vi "Open VIRef in Library App Context.vi"(8 "error in (no error)":errorcluster, 10 "vi path":path, 11 "library in":refnum<vi>) -> (0 "error out":errorcluster, 2 "vi":refnum<vi>, 3 "library out":refnum<vi>)   [LabVIEW 2019, in "gRPC Template Creation Utility.lvlib"]
uses:
  gRPC Template Creation Utility.lvlib
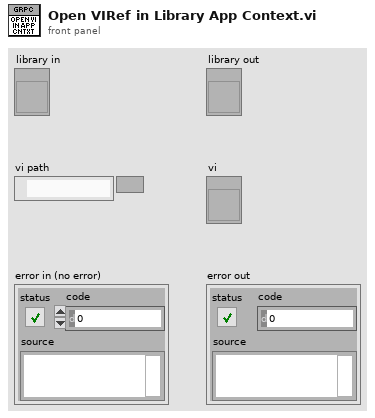
[diagram p1: front panel]
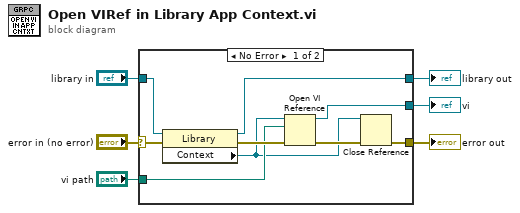
[diagram p0: block diagram]
diagram:
  n1 = case shown="No Error" "error in (no error)" {
    selector: "error in (no error)" -> [w11 w16]
    tunnel: "library in" -> [w12 w17]
    tunnel: [w14 w17] -> w5
    tunnel: [w8 w16] -> w4
    tunnel: [w15 _] -> w2
    tunnel: "vi path" -> [w10 _]
    frame No Error {
      n2 = property class="Library"(reference=w12, error in=w11) -> (reference out=w14:refnum<vi>, error out=w13:errorcluster, "Context"=w7:refnum<vi>)
      n3 = Open VI Reference(application reference (local)=w7, vi path=w10, error in (no error)=w13) -> (vi reference=w15:refnum<vi>, error out=w9:errorcluster)  [unwired: 3 in]
      n4 = Close Reference(reference=w7, error in (no error)=w9) -> (error out=w8:errorcluster)
    }
    frame Error {
    }
  }
  "library out" <- w5
  "error out" <- w4
  "vi" <- w2
